vi "getDataRetrievalMethod.vi"(8 "error in (no error)":errorcluster, 11 "CCD in":refnum<class "CCD.lvclass">) -> (0 "error out":errorcluster, 3 "CCD out":refnum<class "CCD.lvclass">)   [LabVIEW 2023, in "CCD.lvclass"]
uses:
  CCD.lvclass
  CCD.lvclass/CCD.ctl
  20f7d3bd-08ac-4524-9bed-df36c1da25a0.vi
  a21955fc-e3a0-4e36-8495-41f1bfac7860.vi
  GenericDevice/GenericDevice.lvclass
  <vilib>/IlluminatedG/lv-web-crypto/lv-json/JSON/JSON.lvlib
panel:
  # "Connector Pane"
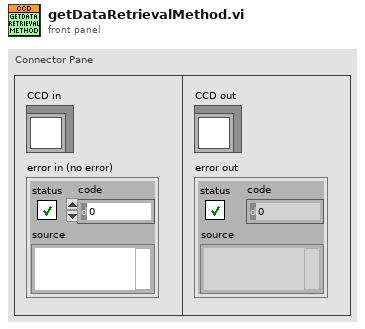
[diagram p1: front panel]
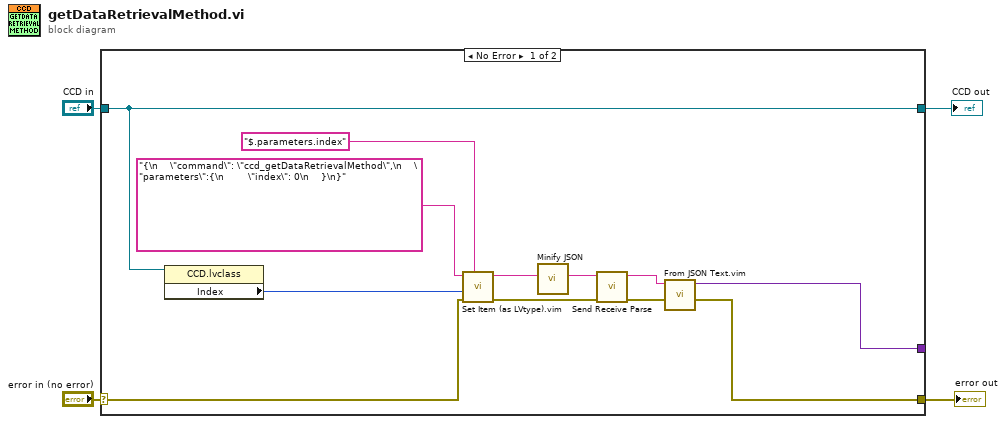
[diagram p0: block diagram]
diagram:
  n1 = case shown="No Error" "error in (no error)" {
    selector: "error in (no error)" -> [w12 w18]
    tunnel: [w10 w18] -> w3
    tunnel: [w14 w17] -> w1
    tunnel: "CCD in" -> [w14 w17]
    tunnel: [w11 _] -> _
    frame No Error {
      n2 = property class="CCD.lvclass"(reference=w14) -> ("Index"=w13:i32)  [unwired: 1 in, 2 out]
      n3 = call "Set Item (as LVtype).vim"("$Path or Item Name"="$.parameters.index", "error in (no error)"=w12, "Anything"=w13, "JSON"="{\n    \"command\": \"ccd_getDataRetrievalMethod\",\n    \"parameters\":{\n        \"index\": 0\n    }\n}") -> ("error out"=w8:errorcluster, "<JSON>"=w6:string)  [unwired: 4 in, 1 out]
      n4 = call <vilib>:"Minify JSON.vi"("JSON String"=w6) -> ("Minified JSON"=w5:string)  [unwired: 10 in]
      n5 = call "Send Receive Parse.vi"("error in"=w8, "<JSON>"=w5) -> ("error out"=w7:errorcluster, "results-JSON string"=w9:string)  [unwired: 7 in, 1 out]
      n6 = call "From JSON Text.vim"("error in (no error)"=w7, "JSON"=w9) -> ("error out"=w10:errorcluster, "Data out"=w11:variant)  [unwired: 8 in]
    }
    frame Error {
    }
  }
  "error out" <- w3
  "CCD out" <- w1
